vi "DrawScoreAndLevel.vi"(8 "error in (no error)":errorcluster, 11 "Bouncer in":refnum<class "Bouncer.lvclass">) -> (0 "error out":errorcluster, 3 "Bouncer out":refnum<class "Bouncer.lvclass">)   [LabVIEW 2019, in "RT_Game.lvlib" / "Bouncer.lvclass"]
uses:
  Bouncer.lvclass
  C:/Users/FreshBob/Dropbox/VIs/myRIO_GameConsole/RT/RT_Game/Game/Game.lvclass
  Game/Coordinate.ctl
  Color.ctl
  Bouncer.lvclass/Bouncer.ctl
  Game/Game.lvclass
  RT_Game.lvlib
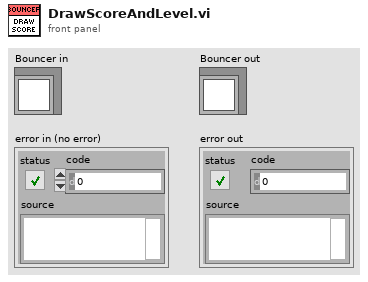
[diagram p1: front panel]
types:
  T1 = typedef "RT_Game.lvlib/Game.lvclass/Coordinate.ctl" = cluster{"x":dbl, "y":dbl}
  T2 = typedef "RT_Game.lvlib/Color.ctl" = fxp<+,3,3>
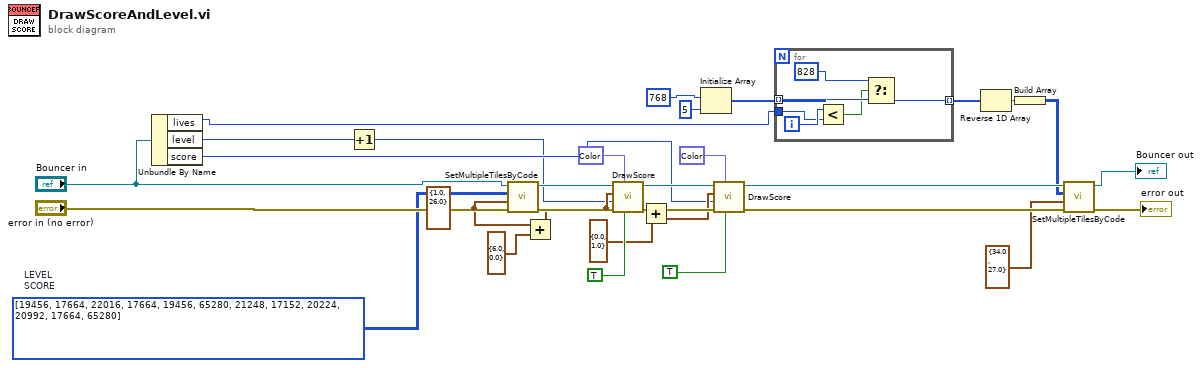
[diagram p0: block diagram]
diagram:
  w23 = T1 {"x"=1.0, "y"=26.0} ("Position")
  w29 = u16[][] [[19456, 17664, 22016, 17664, 19456, 65280], [21248, 17152, 20224, 20992, 17664, 65280]]  # LEVEL  SCORE
  n1 = Unbundle By Name("Bouncer in") -> ("lives"=w7:i16, "level"=w24:i16, "score"=w15:i16)
  n2 = Increment(x=w24) -> (x+1=w1:i16)
  n3 = call "SetMultipleTilesByCode.vi"("error in (no error)"="error in (no error)", "Position"=w23, "TileCodes"=w29, "Game in"="Bouncer in") -> ("error out"=w31:errorcluster, "Game out"=w27:refnum<class "Bouncer.lvclass">)  [unwired: 6 in]
  n4 = Add(x=w23, y=T1 {"x"=6.0, "y"=0.0} ("x")) -> (x+y=w18:T1)
  n5 = call "DrawScore.vi"("AutoWidth?"=TRUE, "Color"=T2 7.0, "error in (no error)"=w31, "score"=w1, "position"=w18, "Pong in"=w27) -> ("error out"=w28:errorcluster, "Pong out"=w20:refnum<class "Bouncer.lvclass">)  [unwired: 4 in]
  n6 = Add(x=w18, y=T1 {"x"=0.0, "y"=1.0} ("x")) -> (x+y=w17:T1)
  n7 = Initialize Array(768 ("Numeric"), 5 ("dimension size")) -> (w8:i32[])
  n8 = call "DrawScore.vi"("AutoWidth?"=TRUE, "Color"=T2 7.0, "error in (no error)"=w28, "score"=w15, "position"=w17, "Pong in"=w20) -> ("error out"=w21:errorcluster, "Pong out"=w12:refnum<class "Bouncer.lvclass">)  [unwired: 4 in]
  n9 = for {
    tunnel: w8 -> [w37] mode=indexing
    tunnel: [w36] -> w6 mode=indexing
    tunnel: w7 -> [w33]
    i -> [w34]
    n10 = Less?(x=w34, y=w33) -> (x < y?=w32:bool)
    n11 = Select(t=828 ("Numeric"), s=w32, f=w37) -> (s? t:f=w36:i32)
  }
  n12 = Reverse 1D Array(array=w6) -> (reversed array=w5:i32[])
  n13 = Build Array(w5) -> (w4:i32[][])
  n14 = call "SetMultipleTilesByCode.vi"("error in (no error)"=w21, "Position"=T1 {"x"=34.0, "y"=27.0}, "TileCodes"=w4, "Game in"=w12) -> ("error out"=→"error out":errorcluster, "Game out"=→"Bouncer out":refnum<class "Bouncer.lvclass">)  [unwired: 6 in]
